vi "Simple PID Array.vi"(8 "D":dbl=0.05 format="%.2f", 9 "I":dbl=0.1 format="%.2f", 10 "P":dbl=1.0 format="%.2f", 11 "process variable":dbl[](array[numeric]) format="%.2f") -> (3 "output value":dbl[](array[numeric]) format="%.2f")   [LabVIEW 2019, in "Instrument.Lockin.lvlib" / "Instrument.DAQ.lvclass"]
uses:
  Instrument.DAQ.lvclass
panel:
  in  "upper limit":dbl=180.0 format="%.2f"
  in  "lower limit":dbl=-180.0 format="%.2f"
  in  "set point":dbl format="%.2f"
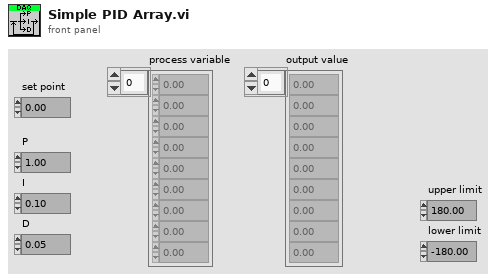
[diagram p1: front panel]
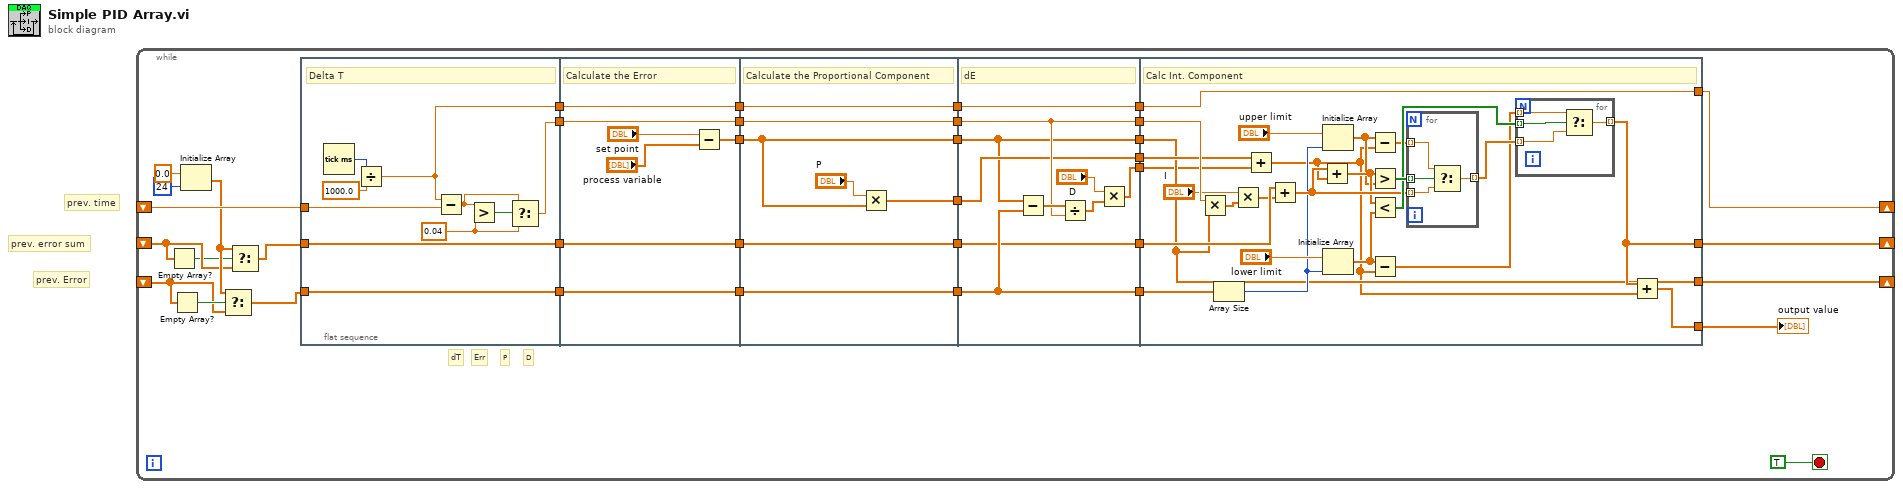
[diagram p0: block diagram]
diagram:
  # "prev. time"
  # "prev. error sum"
  # "prev. Error"
  n1 = while {
    shift-left: _ -> [w29]
    shift-right: [w35] -> _
    shift-left: _ -> [w25]
    shift-right: [w36] -> _
    shift-left: _ -> [w37]
    shift-right: [w1] -> _
    stop <- TRUE stop-if-true
    # "dT"
    # "Err"
    # "D"
    # "P"
    n2 = Empty Array?(array=w25) -> (empty?=w24:bool)
    n3 = Empty Array?(array=w29) -> (empty?=w30:bool)
    n4 = Initialize Array(0.0 ("element"), 24 ("dimension size")) -> (w27:dbl[])
    n5 = Select(t=w27, s=w30, f=w29) -> (s? t:f=w28:dbl[])
    n6 = Select(t=w27, s=w24, f=w25) -> (s? t:f=w26:dbl[])
    n7 = flat-sequence {
      tunnel: [w44] -> w23
      tunnel: w37 -> [w47]
      tunnel: w26 -> [w39]
      tunnel: [w39] -> w22
      tunnel: w28 -> [w38]
      tunnel: [w38] -> w21
      tunnel: [w41] -> w20
      tunnel: w23 -> [w51]
      tunnel: [w51] -> w19
      tunnel: w22 -> [w50]
      tunnel: [w50] -> w18
      tunnel: w21 -> [w49]
      tunnel: [w49] -> w17
      tunnel: w20 -> [w48]
      tunnel: [w48] -> w16
      tunnel: [w53] -> w15
      tunnel: w19 -> [w59]
      tunnel: [w59] -> w14
      tunnel: w18 -> [w58]
      tunnel: [w58] -> w13
      tunnel: w17 -> [w56]
      tunnel: w16 -> [w57]
      tunnel: [w57] -> w12
      tunnel: w15 -> [w55]
      tunnel: [w55] -> w11
      tunnel: [w60] -> w10
      tunnel: [w56] -> w2
      tunnel: w14 -> [w65]
      tunnel: [w65] -> w9
      tunnel: w13 -> [w64]
      tunnel: [w64] -> w8
      tunnel: [w71] -> w7
      tunnel: w12 -> [w66]
      tunnel: [w66] -> w6
      tunnel: w11 -> [w62]
      tunnel: [w62] -> w5
      tunnel: w10 -> [w63]
      tunnel: [w63] -> w4
      tunnel: [w67] -> w3
      tunnel: w2 -> [w71]
      tunnel: [w77] -> w1
      tunnel: w9 -> [w77]
      tunnel: w8 -> [w96]
      tunnel: [w76] -> w36
      tunnel: [w74] -> w35
      tunnel: w7 -> [w75]
      tunnel: [w89] -> w33
      tunnel: w6 -> [w95]
      tunnel: w5 -> [w74]
      tunnel: w4 -> [w91]
      tunnel: w3 -> [w73]
      frame #0 {
        w40 = 0.04
        # "Delta T"
        n8 = Tick Count (ms)() -> (millisecond timer value=w45:u32)
        n9 = Divide(x=w45, y=1000.0) -> (x/y=w44:dbl)
        n10 = Subtract(x=w44, y=w47) -> (x-y=w42:dbl)
        n11 = Greater?(x=w42, y=w40) -> (0:w43:bool)
        n12 = Select(t=w42, s=w43, f=w40) -> (s? t:f=w41:dbl)
      }
      frame #1 {
        # "Calculate the Error"
        n13 = Subtract(x="set point", y="process variable") -> (x-y=w53:dbl[])
      }
      frame #2 {
        # "Calculate the Proportional Component"
        n14 = Multiply(x="P", y=w55) -> (x*y=w60:dbl[])
      }
      frame #3 {
        # "dE"
        n15 = Subtract(x=w62, y=w71) -> (x-y=w70:dbl[])
        n16 = Divide(x=w70, y=w66) -> (x/y=w69:dbl[])
        n17 = Multiply(x="D", y=w69) -> (x*y=w67:dbl[])
      }
      frame #4 {
        # "Calc Int. Component"
        n18 = Multiply(x=w95, y=w74) -> (x*y=w94:dbl[])
        n19 = Array Size(array=w75) -> (size(s)=w78:i32)
        n20 = Multiply(x="I", y=w94) -> (x*y=w92:dbl[])
        n21 = Add(x=w91, y=w73) -> (x+y=w72:dbl[])
        n22 = Add(x=w96, y=w92) -> (x+y=w87:dbl[])
        n23 = Add(x=w87, y=w72) -> (x+y=w85:dbl[])
        n24 = Initialize Array("upper limit", w78) -> (w79:dbl[])
        n25 = Initialize Array("lower limit", w78) -> (w81:dbl[])
        n26 = Subtract(x=w79, y=w72) -> (x-y=w84:dbl[])
        n27 = Greater?(x=w85, y=w79) -> (0:w90:bool[])
        n28 = Less?(x=w85, y=w81) -> (x < y?=w88:bool[])
        n29 = Subtract(x=w81, y=w72) -> (x-y=w83:dbl[])
        n30 = for {
          tunnel: w90 -> [w104] mode=indexing
          tunnel: w87 -> [w103] mode=indexing
          tunnel: [w102] -> w86 mode=indexing
          tunnel: w84 -> [w101] mode=indexing
          n31 = Select(t=w101, s=w104, f=w103) -> (s? t:f=w102:dbl)
        }
        n32 = for {
          tunnel: w88 -> [w100] mode=indexing
          tunnel: w86 -> [w99] mode=indexing
          tunnel: [w98] -> w76 mode=indexing
          tunnel: w83 -> [w97] mode=indexing
          n33 = Select(t=w97, s=w100, f=w99) -> (s? t:f=w98:dbl)
        }
        n34 = Add(x=w76, y=w72) -> (x+y=w89:dbl[])
      }
    }
    "output value" <- w33
  }
